vi "Configure Trigger (Transition).vi"(0 "VISA resource name":refnum<visa-resource-name>, 1 "Time Limit (1E-9 s)":dbl=1e-09, 5 "Trigger Source (1: Channel1)":i32(ring)=1 items=["Channel1"=1, "Channel2"=2, "Channel3"=3, "Channel4"=4], 7 "Violation Mode (0: Greater Than)":i32(ring) items=["Greater Than", "Less Than"], 9 "Trigger Polarity (0: Rising)":i32(ring) items=["Rising", "Falling"], 11 "error in (no error)":errorcluster) -> (4 "VISA resource name out":refnum<visa-resource-name>, 15 "error out":errorcluster)   [LabVIEW 2020, in "Agilent 90000 Series.lvlib"]
doc: "Configures the transition trigger parameters."
uses:
  Agilent 90000 Series.lvlib
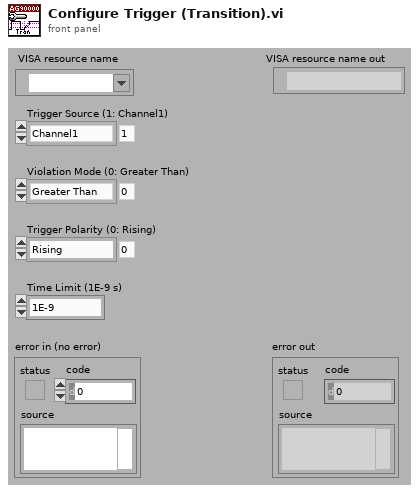
[diagram p1: front panel]
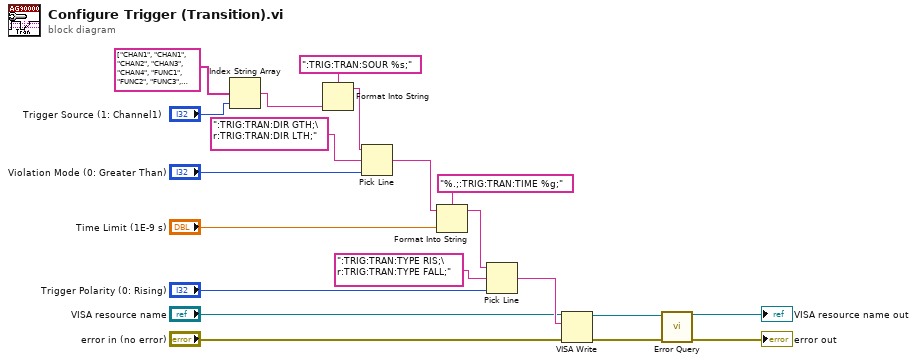
[diagram p0: block diagram]
diagram:
  n1 = Index String Array(1:"Trigger Source (1: Channel1)", 2:string[] ["CHAN1", "CHAN1", "CHAN2", "CHAN3", "CHAN4", "FUNC1", "FUNC2", "FUNC3", "FUNC4", "WMEM1", "WMEM2", "WMEM3", "WMEM4", "AUX", "LINE"]) -> (0:w2:string)  [unwired: 1 out]
  n2 = Format Into String(format string=":TRIG:TRAN:SOUR %s;", w2) -> (resulting string=w1:string)  [unwired: 2 in, 1 out]
  n3 = Pick Line(string ("")=w1, multi-line string=":TRIG:TRAN:DIR GTH;\r:TRIG:TRAN:DIR LTH;", line index="Violation Mode (0: Greater Than)") -> (output string=w18:string)
  n4 = Format Into String(format string="%.;:TRIG:TRAN:TIME %g;", initial string=w18, "Time Limit (1E-9 s)") -> (resulting string=w15:string)  [unwired: 1 in, 1 out]
  n5 = Pick Line(string ("")=w15, multi-line string=":TRIG:TRAN:TYPE RIS;\r:TRIG:TRAN:TYPE FALL;", line index="Trigger Polarity (0: Rising)") -> (output string=w12:string)
  n6 = VISA Write(VISA resource name="VISA resource name", write buffer=w12, error in (no error)="error in (no error)") -> (VISA resource name out=w9:refnum<visa-resource-name>, error out=w8:errorcluster)  [unwired: 1 out]
  n7 = call "Error Query.vi"("error in (no error)"=w8, "VISA resource name"=w9) -> ("error out"=→"error out":errorcluster, "VISA resource name out"=→"VISA resource name out":refnum<visa-resource-name>)  [unwired: 8 out]
